vi "FMDLDiodeConfigKeithley2450SourceVMeasureIMode.vi"(5 "Measurement Speed (NPLC)":dbl=1.0 format="%.2g", 6 "Measurement Count":i32=1 min=1 max=300000 step=1, 7 "Enable High Capacitance (T:Enable)":bool=TRUE, 8 "error in (no error)":errorcluster, 10 "LED bias settings":T1={"Steps (number)"=51, "Vdevice (starting, V)"=0.0, "Vdevice (ending, V)"=5.0, "Accurate readback?"=TRUE, "Current compliance (A)"=0.1} {"Vdevice (ending, V)" min=0.1 max=12.0 step=0.05; "Vdevice (starting, V)" min=0.0 max=20.0 step=0.05; "Steps (number)" min=5 max=1001 step=1}, 11 "VISA resource name in":refnum<visa-resource-name>) -> (0 "error out":errorcluster, 3 "VISA resource name out":refnum<visa-resource-name>)   [LabVIEW 2018]
uses:
  <instrlib>/Keithley 2450/Keithley 2450.lvlib
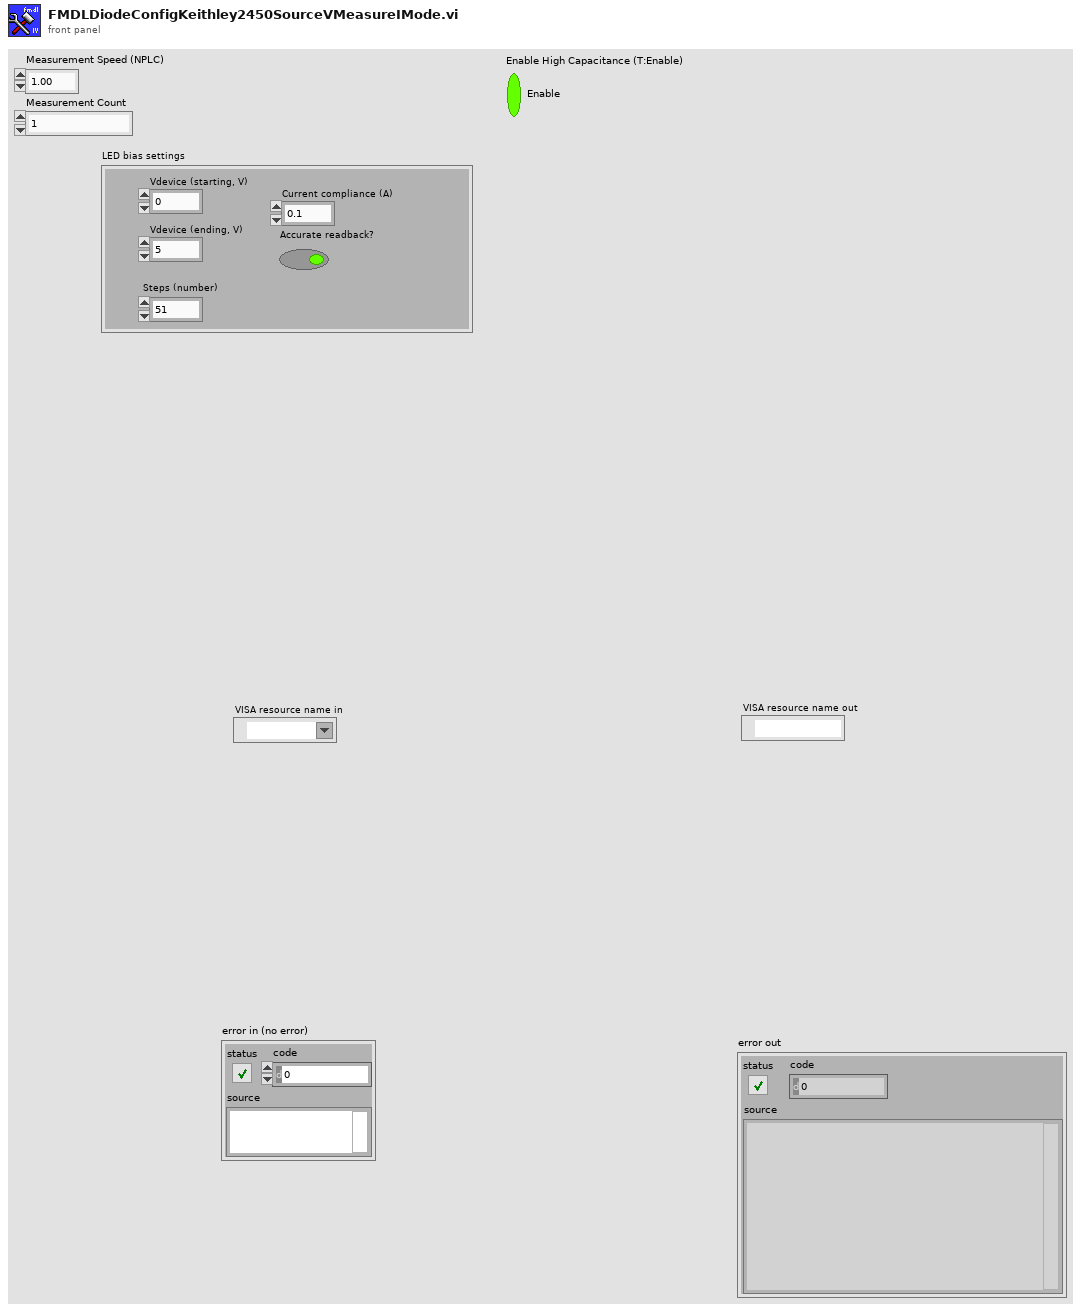
[diagram p1: front panel]
types:
  T1 = cluster{"Steps (number)":i32, "Vdevice (starting, V)":dbl, "Vdevice (ending, V)":dbl, "Accurate readback?":bool, "Current compliance (A)":dbl}
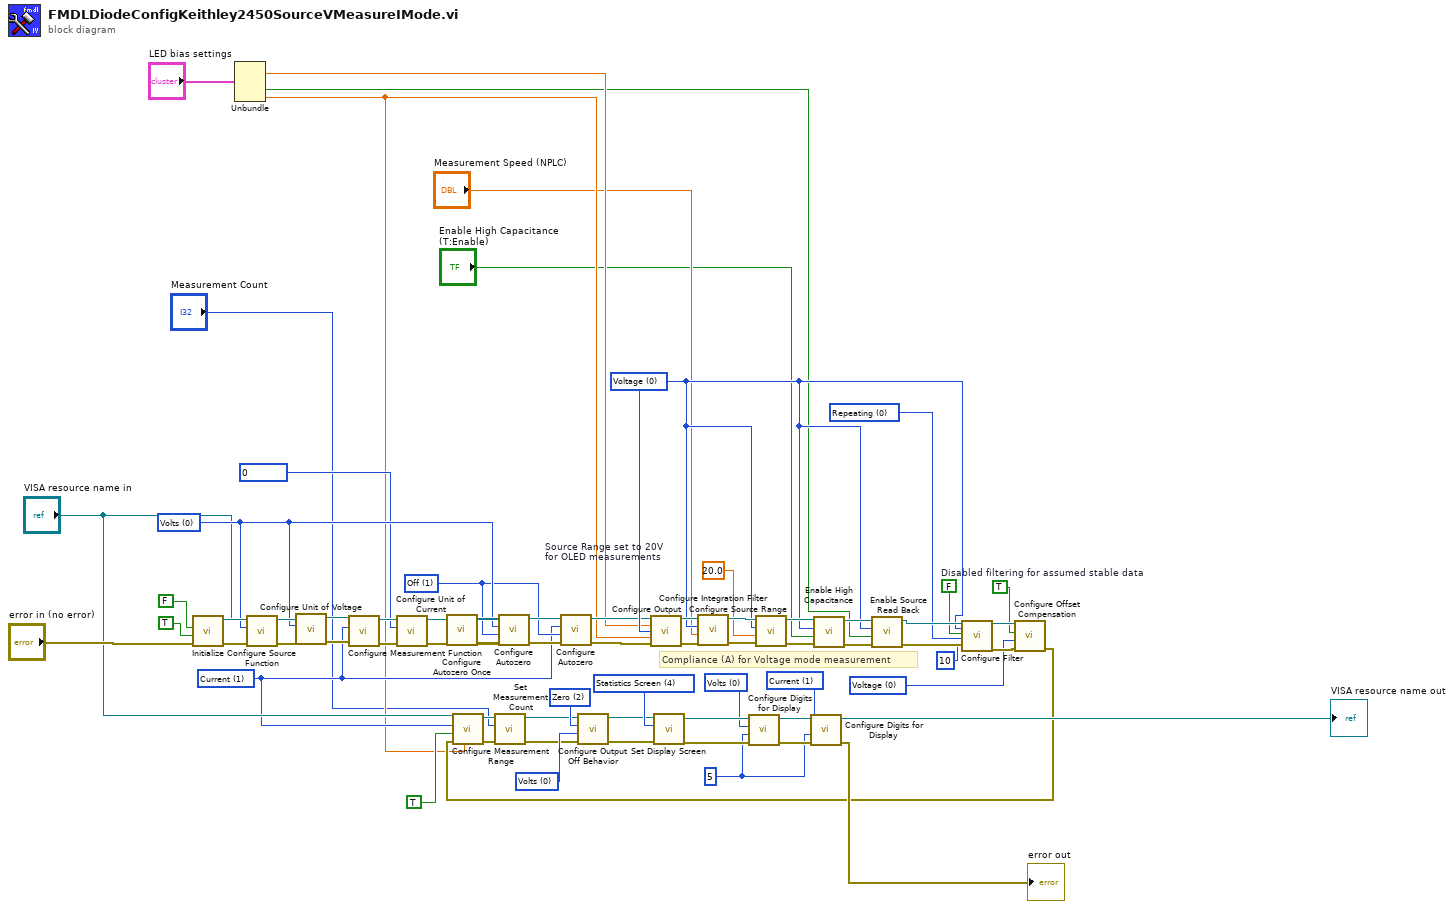
[diagram p0: block diagram]
diagram:
  w11 = u16 1 items=["On", "Off"] ("Autozero  (0: On)")
  w34 = u16 0 items=["Voltage", "Current", "Resistance"] ("Function")
  w39 = u16 1 items=["Volts", "Current", "Resistance", "Digitize Voltage", "Digitize Current"] ("Function (0: Volts)")
  w38 = u32 5 ("Display Digits (3)")
  w42 = u16 0 items=["Volts", "Current", "Resistance", "Digitize Voltage", "Digitize Current"] ("Function (0: Volts)")
  w47 = u16 4 items=["Home Screen", "Source Screen", "Plot Screen", "User-defined Screen", "Statistics Screen", "Settings Screen", "Graph Screen", "Data sheet Screen"] ("Screen Home")
  w48 = u16 0 items=["Volts", "Current"] ("Function (0: Volts)")
  w49 = u16 2 items=["Normal", "High Impedance", "Zero", "Guard"] ("Output Off Behavior (0: Normal)")
  w12 = u16 0 items=["Volts", "Watts", "Ohms"] ("Unit (0: Volts)")
  w8 = u16 1 items=["Volts", "Current", "Auto Resistance", "Manual Resistance", "Digitize Voltage", "Digitize Current"] ("Function (0: Volts)")
  w58 = u16 0 items=["Repeating", "Moving"] ("Filter Type  (0: Repeating)")
  w61 = FALSE  # Disabled filtering for assumed stable data
  w51 = 20.0  # Source Range set to 20V for OLED measurements
  w52 = u16 0 items=["Voltage", "Current"] ("Source Mode  (0: Voltage)")
  # "Compliance (A) for Voltage mode measurement"
  n1 = call <instrlib>:"Initialize.vi"("error in (no error)"="error in (no error)", "Reset (True)"=TRUE, "ID Query (True)"=FALSE, "VISA resource name"="VISA resource name in") -> ("error out"=w24:errorcluster, "VISA resource name out"=w25:refnum<visa-resource-name>)  [unwired: 6 in]
  n2 = Unbundle("LED bias settings") -> ("Vdevice (starting, V)"=w6:dbl, "Accurate readback?"=w4:bool, "Current compliance (A)"=w5:dbl)  [unwired: 2 out]
  n3 = call <instrlib>:"Configure Source Function.vi"("error in (no error)"=w24, "Function (0: Volts)"=w12, "VISA resource name"=w25) -> ("error out"=w22:errorcluster, "VISA resource name out"=w23:refnum<visa-resource-name>)  [unwired: 7 in]
  n4 = call <instrlib>:"Configure Unit of Voltage.vi"("error in (no error)"=w22, "Unit (0: Volts)"=w12, "VISA resource name"=w23) -> ("error out"=w19:errorcluster, "VISA resource name out"=w20:refnum<visa-resource-name>)  [unwired: 7 in]
  n5 = call <instrlib>:"Configure Measurement Function.vi"("error in (no error)"=w19, "Function (0: Volts)"=w8, "VISA resource name"=w20) -> ("error out"=w17:errorcluster, "VISA resource name out"=w18:refnum<visa-resource-name>)  [unwired: 7 in]
  n6 = call <instrlib>:"Configure Unit of Current.vi"("error in (no error)"=w17, "Unit (0: Amps)"=u16 0, "VISA resource name"=w18) -> ("error out"=w54:errorcluster, "VISA resource name out"=w55:refnum<visa-resource-name>)  [unwired: 7 in]
  n7 = call <instrlib>:"Configure Autozero Once.vi"("error in (no error)"=w54, "VISA resource name"=w55) -> ("error out"=w26:errorcluster, "VISA resource name out"=w27:refnum<visa-resource-name>)  [unwired: 8 in]
  n8 = call <instrlib>:"Configure Autozero.vi"("error in (no error)"=w26, "Autozero  (0: On)"=w11, "Function (0: Volts)"=w12, "VISA resource name"=w27) -> ("error out"=w15:errorcluster, "VISA resource name out"=w16:refnum<visa-resource-name>)  [unwired: 6 in]
  n9 = call <instrlib>:"Configure Autozero.vi"("error in (no error)"=w15, "Autozero  (0: On)"=w11, "Function (0: Volts)"=w8, "VISA resource name"=w16) -> ("error out"=w13:errorcluster, "VISA resource name out"=w14:refnum<visa-resource-name>)  [unwired: 6 in]
  n10 = call <instrlib>:"Configure Output.vi"("VISA resource name"=w14, "Source Level (0)"=w6, "Source Mode  (0: Voltage)"=w52, "Source Limit Level (0.1)"=w5, "error in (no error)"=w13) -> ("VISA resource name out"=w70:refnum<visa-resource-name>, "error out"=w69:errorcluster)  [unwired: 9 in]
  n11 = call <instrlib>:"Configure Integration Filter.vi"("error in (no error)"=w69, "Measurement Speed (1 PLC)"="Measurement Speed (NPLC)", "Function (0: Volts)"=w52, "VISA resource name"=w70) -> ("error out"=w67:errorcluster, "VISA resource name out"=w68:refnum<visa-resource-name>)  [unwired: 6 in]
  n12 = call <instrlib>:"Configure Source Range.vi"("error in (no error)"=w67, "Source Range (1.0)"=w51, "Function (0: Volts)"=w52, "VISA resource name"=w68) -> ("error out"=w65:errorcluster, "VISA resource name out"=w66:refnum<visa-resource-name>)  [unwired: 6 in]
  n13 = call <instrlib>:"Enable High Capacitance.vi"("error in (no error)"=w65, "Enable High Capacitance (T:Enable)"="Enable High Capacitance (T:Enable)", "Function (0: Volts)"=w52, "VISA resource name"=w66) -> ("error out"=w63:errorcluster, "VISA resource name out"=w64:refnum<visa-resource-name>)  [unwired: 6 in]
  n14 = call <instrlib>:"Enable Source Read Back.vi"("error in (no error)"=w63, "Enable Read Back  (T:Enable)"=w4, "Function (0: Volts)"=w52, "VISA resource name"=w64) -> ("error out"=w60:errorcluster, "VISA resource name out"=w62:refnum<visa-resource-name>)  [unwired: 6 in]
  n15 = call <instrlib>:"Configure Filter.vi"("VISA resource name"=w62, "Function (0: Volts)"=w52, "Enable Filter  (T: Enable)"=w61, "Filter Type  (0: Repeating)"=w58, "Number of Filter Readings (3)"=u32 10, "error in (no error)"=w60) -> ("VISA resource name out"=w37:refnum<visa-resource-name>, "error out"=w36:errorcluster)  [unwired: 12 in]
  n16 = call <instrlib>:"Configure Offset Compensation.vi"("error in (no error)"=w36, "Function"=w34, "Enable Compensation (T: Enable)"=TRUE, "VISA resource name"=w37) -> ("error out"=w21:errorcluster)  [unwired: 6 in, 1 out]
  n17 = call <instrlib>:"Configure Measurement Range.vi"("Manual Range (1.0)"=w5, "error in (no error)"=w21, "Enable Auto Range (T:Enable)"=TRUE, "Function (0: Volts)"=w8, "VISA resource name"="VISA resource name in") -> ("error out"=w32:errorcluster, "VISA resource name out"=w33:refnum<visa-resource-name>)  [unwired: 5 in]
  n18 = call <instrlib>:"Set Measurement Count.vi"("error in (no error)"=w32, "Measurement Count"="Measurement Count", "VISA resource name"=w33) -> ("error out"=w30:errorcluster, "VISA resource name out"=w31:refnum<visa-resource-name>)  [unwired: 7 in]
  n19 = call <instrlib>:"Configure Output Off Behavior.vi"("error in (no error)"=w30, "Function (0: Volts)"=w48, "Output Off Behavior (0: Normal)"=w49, "VISA resource name"=w31) -> ("error out"=w45:errorcluster, "VISA resource name out"=w46:refnum<visa-resource-name>)  [unwired: 6 in]
  n20 = call <instrlib>:"Set Display Screen.vi"("error in (no error)"=w45, "Screen Home"=w47, "VISA resource name"=w46) -> ("error out"=w44:errorcluster, "VISA resource name out"=w43:refnum<visa-resource-name>)  [unwired: 7 in]
  n21 = call <instrlib>:"Configure Digits for Display.vi"("error in (no error)"=w44, "Display Digits (3)"=w38, "Function (0: Volts)"=w42, "VISA resource name"=w43) -> ("error out"=w40:errorcluster, "VISA resource name out"=w41:refnum<visa-resource-name>)  [unwired: 6 in]
  n22 = call <instrlib>:"Configure Digits for Display.vi"("error in (no error)"=w40, "Display Digits (3)"=w38, "Function (0: Volts)"=w39, "VISA resource name"=w41) -> ("error out"=→"error out":errorcluster, "VISA resource name out"=→"VISA resource name out":refnum<visa-resource-name>)  [unwired: 6 in]
